vi "AMC QR Add Queue .vi"(8 "error in (no error)":errorcluster, 10 "Name":string, 11 "Message Queue in":T1) -> (0 "error out":errorcluster, 3 "Message Queue out":T1)   [LabVIEW 2017]
doc: "This VI removes the host connection from the connection manager list if it becomes disconnected for any reason."
uses:
  subVIs/TypeDefs/amc_Message Queue.ctl
  subVIs/TypeDefs/amc_Message.ctl
  Tools/Keyed Array/Tools_KeyedArray KeyedArray.ctl
  TypeDefs/amc_QueueRegistryMethod.ctl
  TypeDefs/amc_QueueRegistryProperties.ctl
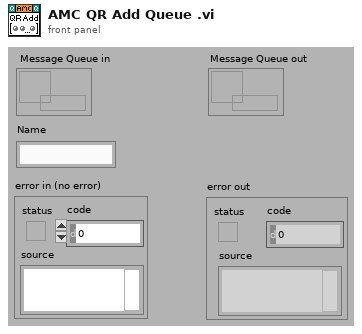
[diagram p1: front panel]
types:
  T1 = typedef "amc_Message Queue.ctl" = refnum<queue>
  T2 = typedef "amc_QueueRegistryProperties.ctl" = cluster{"Name":string}
  T3 = typedef "amc_QueueRegistryMethod.ctl" = enum16{"Initialize", "Add Queue", "Set Properties", "Get Queue by Index", "Get Queue by Name", "Remove Queue", "Remove All Queues"}
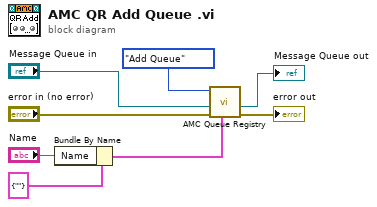
[diagram p0: block diagram]
diagram:
  n1 = Bundle By Name(cluster=T2 {"Name"=""} ("Properties In"), "Name"="Name") -> (w5:T2)
  n2 = call "AMC Queue Registry.vi"("Properties in"=w5, "error in (no error)"="error in (no error)", "Message Queue in"="Message Queue in", "Method"=amc_QueueRegistryMethod."Add Queue") -> ("error out"=→"error out":errorcluster, "Message Queue out"=→"Message Queue out":T1)  [unwired: 1 in, 5 out]
